vi "2 PureWaypointHeadingGoodness.vi"(3 "Waypoint Location":T1 {"North" format="%#_10f"; "East" format="%#_8f"}, 4 "Heading to Test":dbl) -> (1 "Goodness":dbl)   [LabVIEW 2011]
doc: "Takes the absolute wind vector, the heading of your next waypoint, and a test heading and outputs a goodness value for the test heading. The criteria is the speed to get to the waypoint.\n\nThe goodness is evaluated by taking the softmax of an angle with all possible complimenting angles (i.e. if the test heading is 10 degrees it is matched with -1 through -89; note that angles are adjusted to be degrees from directly at the waypoint). The specific calculation for finding the net velocity of a pair of angles requires the velocities from the polar plot."
uses:
  2 Typedefs/UTM Location.ctl
  2 Globals/2 Global.vi
panel:
  out "Heading to Waypt":dbl
  # "Inputs"
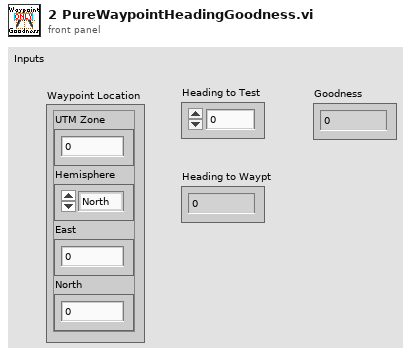
[diagram p1: front panel]
types:
  T1 = typedef "UTM Location.ctl" = cluster{"UTM Zone":dbl, "Hemisphere":enum16{"North", "South"}, "East":dbl, "North":dbl}
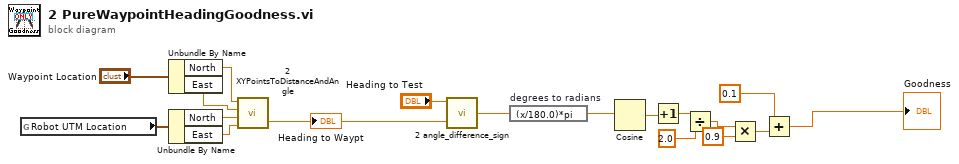
[diagram p0: block diagram]
diagram:
  n1 = global read "2 Global.vi" "Robot UTM Location"() -> (w13:T1)
  n2 = Unbundle By Name("Waypoint Location") -> ("North"=w15:dbl, "East"=w14:dbl)
  n3 = Unbundle By Name(w13) -> ("North"=w16:dbl, "East"=w17:dbl)
  n4 = call "2 XYPointsToDistanceAndAngle.vi"("East 2"=w17, "North 2"=w16, "East 1"=w14, "North 1"=w15) -> ("Angle Diff"=w11:dbl)  [unwired: 1 out]
  "Heading to Waypt" <- w11
  n5 = call "2 angle_difference_sign.vi"("Angle 2"=w11, "Angle 1"="Heading to Test") -> ("Difference"=w9:dbl)
  n6 = expression code="(x/180.0)*pi" "degrees to radians"(w9) -> (w10:dbl)
  n7 = Cosine(x=w10) -> (cos(x)=w8:dbl)
  n8 = Increment(x=w8) -> (x+1=w7:dbl)
  n9 = Divide(x=w7, y=2.0) -> (x/y=w5:dbl)
  n10 = Multiply(x=w5, y=0.9) -> (x*y=w3:dbl)
  n11 = Add(x=0.1, y=w3) -> (x+y=→"Goodness":dbl)
